vi "Teleop.vi"(10 "Match Info":T1={"Autonomous Elapsed Seconds"=0.0, "TeleOp Elapsed Seconds"=0.0, "Disabled Elapsed Seconds"=0.0, "Visited Autonomous"=FALSE, "Visited TeleOp"=FALSE, "Visited Disabled"=FALSE, "Autonomous Settings"={"Autonomous Style"=enum."Independent", "VI Refnum"=refnum}}, 11 "Call Context":T2) -> ()   [LabVIEW 2013]
doc: "This VI is called for each TeleOp packet received from the DS where the robot is not disabled. It is often used to read from the joysticks and update I/O or to update setpoints for timed control loops. It should complete and return within 20 milliseconds or it may miss DS packets."
uses:
  <vilib>/Rock Robotics/WPI/DriverStation/WPI_DriverStationDerivedRobotMode.ctl
  <vilib>/Rock Robotics/WPI/DriverStation/WPI_DriverStationMatch Info.ctl
  RefnameEnum.ctl
  Robot Global Data.vi
  <vilib>/Rock Robotics/WPI/Joystick/WPI_JoystickGetSetRefNum.vi
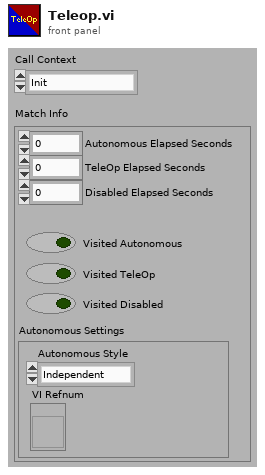
[diagram p1: front panel]
types:
  T1 = typedef "WPI_DriverStationMatch Info.ctl" = cluster{"Autonomous Elapsed Seconds":dbl, "TeleOp Elapsed Seconds":dbl, "Disabled Elapsed Seconds":dbl, "Visited Autonomous":bool, "Visited TeleOp":bool, "Visited Disabled":bool, "Autonomous Settings":cluster{"Autonomous Style":enum16{"Iterative", "Independent"}, "VI Refnum":refnum<vi>}}
  T2 = typedef "WPI_DriverStationDerivedRobotMode.ctl" = enum16{"Init", "Execute", "Stop"}
  T3 = typedef "RefnameEnum.ctl" = enum16{"TankDrive", "Controller1", "Controller2", "SonicShifter", "Compressor"}
  T4 = typedef "WPI_JoystickDevRef.ctl" = cluster{"Device":T5}
  T5 = typedef "WPI_JoystickDeviceEnum.ctl" = enum16{"USB 1", "USB 2", "USB 3", "USB 4", "Kinect 1", "Kinect 2"}
  T6 = typedef "WPI_JoystickButtonState.ctl" = cluster{"Button 1":bool, "Button 2":bool, "Button 3":bool, "Button 4":bool, "Button 5":bool, "Button 6":bool, "Button 7":bool, "Button 8":bool, "Button 9":bool, "Button 10":bool, "Button 11":bool, "Button 12":bool}
  T7 = cluster{"axis 1 (x)":dbl, "axis 2 (y)":dbl, "axis 3 (throttle)":dbl, "axis 4":dbl, "axis 5":dbl, "axis 6":dbl}
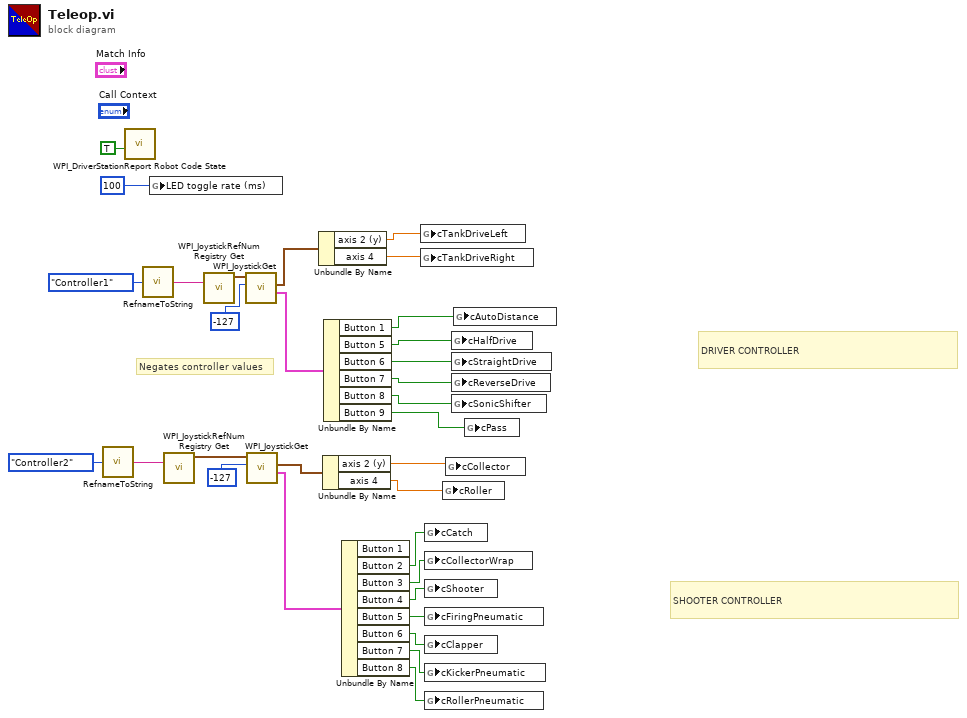
[diagram p0: block diagram]
diagram:
  # "SHOOTER CONTROLLER"
  # "DRIVER CONTROLLER"
  # "Negates controller values"
  n1 = call "RefnameToString.vi"("Enum"=RefnameEnum."Controller2") -> ("Refname"=w16:string)
  n2 = call <vilib>:"WPI_DriverStationReport Robot Code State.vi"("TeleOp"=TRUE ("Autonomous")) -> ()  [unwired: 10 in, 1 out]
  n3 = call "RefnameToString.vi"("Enum"=RefnameEnum."Controller1") -> ("Refname"=w27:string)
  n4 = global write "Robot Global Data.vi" "LED toggle rate (ms)"(u32 100 ("LED ms toggle rate")) -> ()
  n5 = call <vilib>:"WPI_JoystickRefNum Registry Get.vi"("refnum name"=w16) -> ("JoystickDevRef"=w14:T4)  [unwired: 1 in, 9 out]
  n6 = call <vilib>:"WPI_JoystickRefNum Registry Get.vi"("refnum name"=w27) -> ("JoystickDevRef"=w29:T4)  [unwired: 1 in, 9 out]
  n7 = call <vilib>:"WPI_JoystickGet.vi"("Scaler"=i8 -127, "JoystickDevRef"=w29) -> ("Buttons"=w24:T6, "Axes"=w25:T7)  [unwired: 4 out]
  n8 = call <vilib>:"WPI_JoystickGet.vi"("Scaler"=i8 -127, "JoystickDevRef"=w14) -> ("Buttons"=w12:T6, "Axes"=w13:T7)  [unwired: 4 out]
  n9 = Unbundle By Name(w25) -> ("axis 2 (y)"=w22:dbl, "axis 4"=w23:dbl)
  n10 = Unbundle By Name(w13) -> ("axis 2 (y)"=w3:dbl, "axis 4"=w2:dbl)
  n11 = Unbundle By Name(w24) -> ("Button 1"=w4:bool, "Button 5"=w21:bool, "Button 6"=w20:bool, "Button 7"=w18:bool, "Button 8"=w19:bool, "Button 9"=w1:bool)
  n12 = Unbundle By Name(w12) -> ("Button 2"=w6:bool, "Button 3"=w7:bool, "Button 4"=w8:bool, "Button 5"=w5:bool, "Button 6"=w11:bool, "Button 7"=w10:bool, "Button 8"=w9:bool)  [unwired: 1 out]
  n13 = global write "Robot Global Data.vi" "cTankDriveLeft"(w22) -> ()
  n14 = global write "Robot Global Data.vi" "cTankDriveRight"(w23) -> ()
  n15 = global write "Robot Global Data.vi" "cCatch"(w6) -> ()
  n16 = global write "Robot Global Data.vi" "cCollectorWrap"(w7) -> ()
  n17 = global write "Robot Global Data.vi" "cShooter"(w8) -> ()
  n18 = global write "Robot Global Data.vi" "cFiringPneumatic"(w5) -> ()
  n19 = global write "Robot Global Data.vi" "cClapper"(w11) -> ()
  n20 = global write "Robot Global Data.vi" "cKickerPneumatic"(w10) -> ()
  n21 = global write "Robot Global Data.vi" "cRollerPneumatic"(w9) -> ()
  n22 = global write "Robot Global Data.vi" "cRoller"(w2) -> ()
  n23 = global write "Robot Global Data.vi" "cCollector"(w3) -> ()
  n24 = global write "Robot Global Data.vi" "cHalfDrive"(w21) -> ()
  n25 = global write "Robot Global Data.vi" "cStraightDrive"(w20) -> ()
  n26 = global write "Robot Global Data.vi" "cReverseDrive"(w18) -> ()
  n27 = global write "Robot Global Data.vi" "cSonicShifter"(w19) -> ()
  n28 = global write "Robot Global Data.vi" "cAutoDistance"(w4) -> ()
  n29 = global write "Robot Global Data.vi" "cPass"(w1) -> ()
